vi "autosize.vi"(8 "error in (no error)":errorcluster, 10 "Table in":refnum<vi>, 11 "State":T1={"logTable"=refnum, "max items"=500, "displaydata"=[], "data"=[], "Auto Scroll"=TRUE, "current item"=500, "col headers"=[], "Add to Top"=TRUE, "Auto resize"=TRUE, "col size"=[], "filters"=[], "color cells"=[]}) -> (0 "error out":errorcluster, 2 "Table out":refnum<vi>, 3 "State (dup)":T1={"logTable"=refnum, "max items"=500, "displaydata"=[], "data"=[], "Auto Scroll"=TRUE, "current item"=500, "col headers"=[], "Add to Top"=TRUE, "Auto resize"=TRUE, "col size"=[], "filters"=[], "color cells"=[]})   [LabVIEW 2013, in "UI-DisplayTable(dev).xctl"]
uses:
  UI-DisplayTable(dev).xctl
  State.ctl
  DEF-Filter.ctl
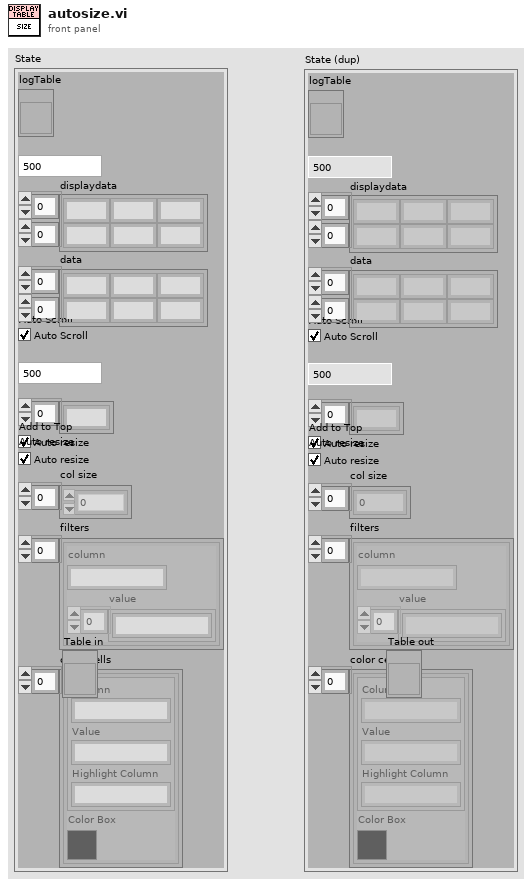
[diagram p1: front panel]
types:
  T1 = typedef "UI-DisplayTable(dev).xctl/State.ctl" = cluster{"logTable":refnum<vi>, "max items":i32, "displaydata":string[][], "data":string[][], "Auto Scroll":bool, "current item":i32, "col headers":string[], "Add to Top":bool, "Auto resize":bool, "col size":i32[], "filters":T2[], "color cells":cluster{"color cell":cluster{"Column":string, "Value":string, "Highlight Column":string}, "Color Box":u32}[]}
  T2 = typedef "UI-DisplayTable(dev).xctl/DEF-Filter.ctl" = cluster{"column":string, "value":string[]}
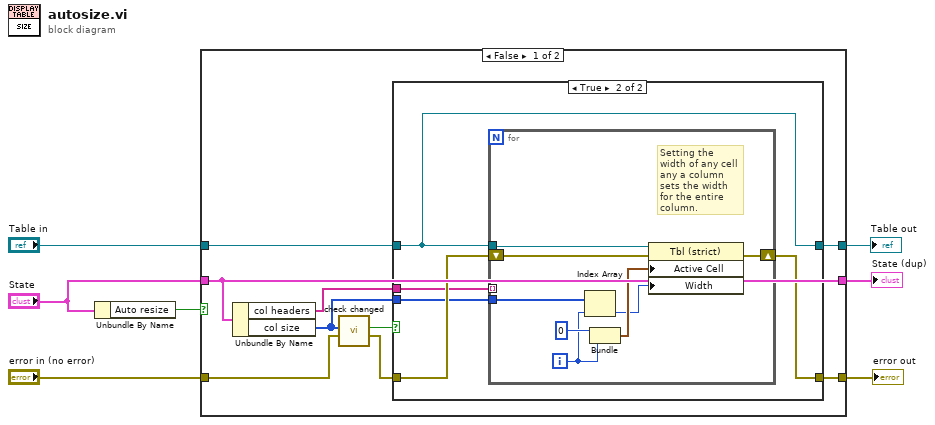
[diagram p0: block diagram]
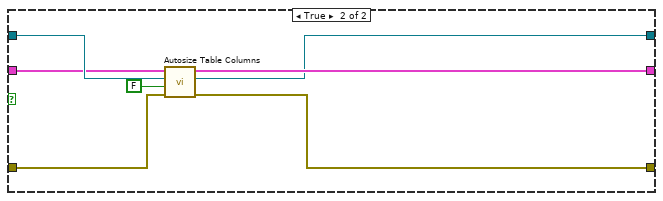
[diagram p3: hidden frame]
diagram:
  n1 = Unbundle By Name("State") -> ("Auto resize"=w7:bool)
  n2 = case shown="False" w7 {
    tunnel: "Table in" -> [w13 w38]
    tunnel: [w12 w35] -> w5
    tunnel: "State" -> [w16 w33]
    tunnel: [w16 w36] -> w3
    tunnel: "error in (no error)" -> [w11 w32]
    tunnel: [w9 w34] -> w1
    frame False {
      n3 = Unbundle By Name(w16) -> ("col headers"=w8:string[], "col size"=w14:i32[])
      n4 = call "check changed.vi"("error in (no error)"=w11, "data"=w14) -> ("error out"=w10:errorcluster, "changed?"=w15:bool)  [unwired: 8 in]
      n5 = case shown="True" w15 {
        tunnel: w14 -> [_ w20]
        tunnel: w13 -> [w18 w23]
        tunnel: [w18 w23] -> w12
        tunnel: w10 -> [w17 w22]
        tunnel: [w17 w21] -> w9
        tunnel: w8 -> [_ w19]
        frame False {
        }
        frame True {
          n6 = for {
            tunnel: w23 -> [w30]
            shift-right: [w28] -> w21
            shift-left: w22 -> [w29]
            tunnel: w20 -> [w26]
            tunnel: w19 -> [_] mode=indexing
            i -> [w25]
            # "Setting the width of any cell any a column sets the width for the entire column."
            n7 = Index Array(array=w26, index=w25) -> (element=w24:i32)
            n8 = Bundle(0, w25) -> (w31:cluster{i32, i32})  [unwired: 1 in]
            n9 = property class="Tbl (strict)"(reference=w30, error in=w29, "Active Cell"=w31, "Width"=w24) -> (error out=w28:errorcluster)  [unwired: 1 out]
          }
        }
      }
    }
    frame True {
      n10 = call "Autosize Table Columns.vi"("error in (no error)"=w32, "Resize Table?"=FALSE, "Table Ref"=w38, "State"=w33) -> ("error out"=w34:errorcluster, "Table Ref (dup)"=w35:refnum<vi>, "State (dup)"=w36:T1)  [unwired: 5 in]
    }
  }
  "error out" <- w1
  "State (dup)" <- w3
  "Table out" <- w5
